vi "Unpack Acquisition Result.vi"(8 "Error In":errorcluster, 9 "Acquisition Results":T1[](array[typedef]) {"Update rate [1/s]" format="%_3p"}, 10 "Averaging":T2 {"Traces" min=1 max=200 step=1}) -> (0 "Error Out":errorcluster, 1 "Last Acquisition Result":T1={"Traces"=[], "Relative t0 [s]"=1000.0, "Sample Rate [1/s]"=1000.0, "No. of points"=0, "Absolute t0 [s]"=1000.0, "dT [s]"=1000.0, "Update rate [1/s]"=0.0, "Auto Triggered"=FALSE, "Stop"=FALSE} {"Update rate [1/s]" format="%_3p"}, 2 "Traces":waveform(dbl)[][](array[waveform]))   [LabVIEW 2019]
uses:
  Averaging.ctl
  Controls/Acquisition Result.ctl
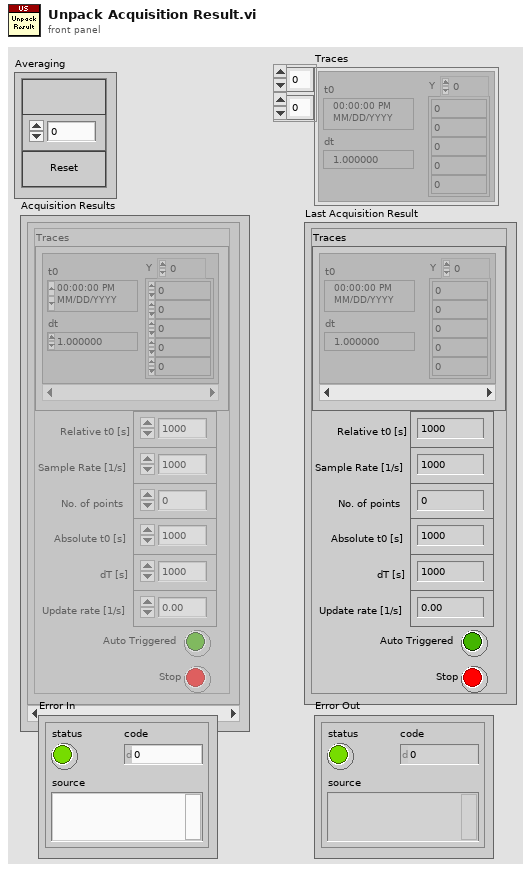
[diagram p1: front panel]
types:
  T1 = typedef "Acquisition Result.ctl" = cluster{"Traces":waveform(sgl)[], "Relative t0 [s]":dbl, "Sample Rate [1/s]":dbl, "No. of points":i32, "Absolute t0 [s]":dbl, "dT [s]":dbl, "Update rate [1/s]":dbl, "Auto Triggered":bool, "Stop":bool}
  T2 = typedef "Averaging.ctl" = cluster{"On":bool, "Traces":i32, "Reset":bool}
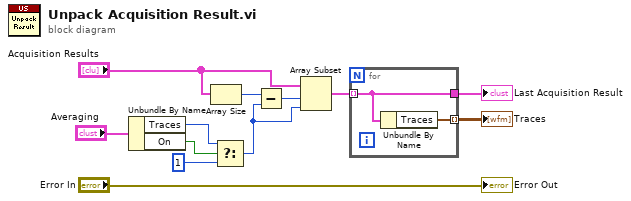
[diagram p0: block diagram]
diagram:
  n1 = Unbundle By Name("Averaging") -> ("Traces"=w9:i32, "On"=w12:bool)
  n2 = Array Size(array="Acquisition Results") -> (size(s)=w7:i32)
  n3 = Select(t=w9, s=w12, f=1) -> (s? t:f=w10:i32)
  n4 = Subtract(x=w7, y=w10) -> (x-y=w8:i32)
  n5 = Array Subset(array="Acquisition Results", index=w8, length=w10) -> (w3:T1[])
  n6 = for {
    tunnel: w3 -> [w13] mode=indexing
    tunnel: [w14] -> w4 mode=indexing
    tunnel: [w13] -> w2
    n7 = Unbundle By Name(w13) -> ("Traces"=w14:waveform(sgl)[])
  }
  "Traces" <- w4
  "Last Acquisition Result" <- w2
  "Error Out" <- "Error In"
